vi "Untitled 1.vi"() -> ()   [LabVIEW 2020]
uses:
  <vilib>/imath/engines/lvmath2/RunTimeEngine/Managers/WorkSpace/UID Generator.vi
  <vilib>/imath/engines/lvmath2/RunTimeEngine/RunTimeType/NIMS_RunTimeType_From StrictType (excl LVString).vi
  <instcachedir>/0/NIMS_RunTimeType_From StrictType (excl LVString)_283B1B2000484AAA8744D21CE97EA49F.lvgen/NIMS_RunTimeType_From StrictType (excl LVString)_283B1B2000484AAA8744D21CE97EA49F_000.vi
  <vilib>/imath/engines/lvmath2/RunTimeEngine/LocalVariableDefStatement/MC_LocalVariableDefStatement_Display.vi
  <vilib>/imath/engines/lvmath2/RunTimeEngine/Managers/SymbolTable/Clear UID.vi
  <vilib>/imath/engines/lvmath2/RunTimeEngine/NodeEndStatement/NIMS_NodeEndStatement_Output.vi
  <instcachedir>/0/NIMS_NodeEndStatement_Output_53EC0D466D134D7ABD903AC30B43404B.lvgen/NIMS_NodeEndStatement_Output_53EC0D466D134D7ABD903AC30B43404B_009.vi
  <vilib>/imath/engines/lvmath2/RunTimeEngine/ErrorHandling/NIMS_Finalize Error.vi
  <vilib>/imath/engines/lvmath2/RunTimeEngine/ArithmeticOperatorToken/NIMS_ArithmeticOperator_power(S).vi
  <instcachedir>/0/NIMS_ArithmeticOperator_power(S)_0FB4C2FA3CD746849DC4699515FAC284.lvgen/NIMS_ArithmeticOperator_power(S)_0FB4C2FA3CD746849DC4699515FAC284_014.vi
  <instcachedir>/0/NIMS_ArithmeticOperator_power(S)_0FB4C2FA3CD746849DC4699515FAC284.lvgen/NIMS_ArithmeticOperator_power(S)_0FB4C2FA3CD746849DC4699515FAC284_010.vi
  <vilib>/imath/engines/lvmath2/RunTimeEngine/ErrorHandling/NIMS_Create Error From Enums.vi
  <vilib>/imath/engines/lvmath2/RunTimeEngine/Managers/SymbolTable/NIMS_WorkSpace.lvlib
panel:
  out "Waveform Graph 2":dbl[](graph)
  in  "n":dbl
  out "Waveform Graph":dbl[](graph)
  in  "a":dbl
  in  "stop":bool
  # "V=sqrt(1/(1-a+(a/(e^(n*(h-1)))^2)))"
  # "h=(2*n-log((-1 + a + 1/V^2)/a))/(2*n)"
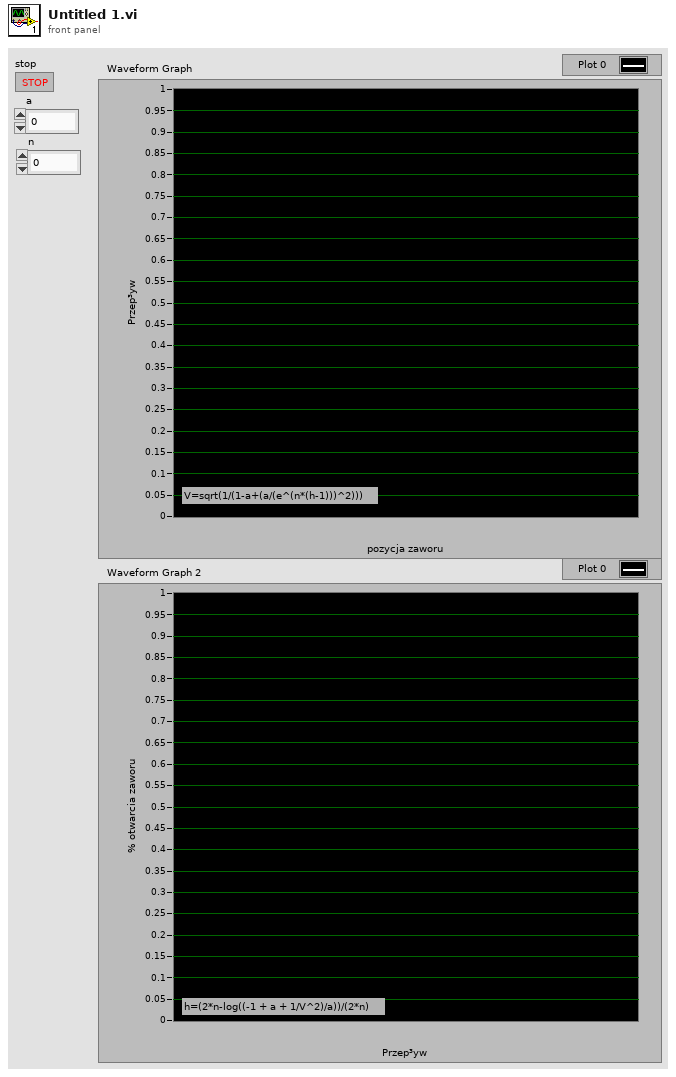
[diagram p1: front panel]
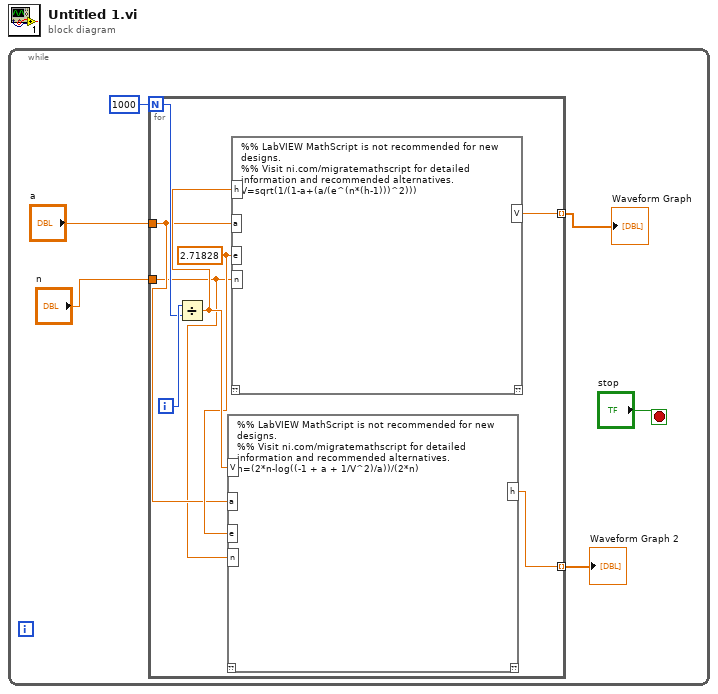
[diagram p0: block diagram]
diagram:
  n1 = while {
    stop <- "stop" stop-if-true
    n2 = for {
      N: 1000 -> [w12]
      tunnel: [w14] -> w4 mode=indexing
      tunnel: "a" -> [w9]
      tunnel: "n" -> [w8]
      tunnel: [w7] -> w1 mode=indexing
      i -> [w13]
      w10 = 2.71828 ("e")
      n3 = Divide(x=w13, y=w12) -> (x/y=w11:dbl)
      n4 = mathscript code="%% LabVIEW MathScript is not recommended for new designs.\n%% Visit ni.com/migratemathscript for detailed information and recommended alternatives.\nh=(2*n-log((-1 + a + 1/V^2)/a))/(2*n)"("V"=w11, "a"=w9, "e"=w10, "n"=w8) -> ("h"=w7:cdb)  [unwired: 1 in, 1 out]
      n5 = mathscript code="%% LabVIEW MathScript is not recommended for new designs.\n%% Visit ni.com/migratemathscript for detailed information and recommended alternatives.\nV=sqrt(1/(1-a+(a/(e^(n*(h-1)))^2)))"("h"=w11, "a"=w9, "e"=w10, "n"=w8) -> ("V"=w14:cdb)  [unwired: 1 in, 1 out]
    }
    "Waveform Graph" <- w4
    "Waveform Graph 2" <- w1
  }
